vi "PPG_ABC.calc temp pattern.vi"(0 "i ref in":refnum<vi>, 2 "PGData":T3, 4 "clockRate [ticks/us]":dbl, 5 "error in (no error)":errorcluster) -> (14 "i ref out":refnum<vi>, 16 "patternDefs":T2(array[cluster]), 19 "error out":errorcluster)   [LabVIEW 2014, in "PPG_ABC.lvlib"]
doc: "Calculates the pattern definition array. This method starts from a public pattern format defined by this class and converts it into an intermediate pattern definition array."
uses:
  PPG_ABC.lvlib
  PPG_ABC.PG_dataType.ctl
  CS_Core/CSSystem/CoreDefs/CoreDefs.error_type.ctl
  CS_Core/CSSystem/CoreDefs/CoreDefs.error_severity.ctl
  CS_Core/CSSystem/CoreLib/CoreLib.lvlib
panel:
  in  "patternDef":T1
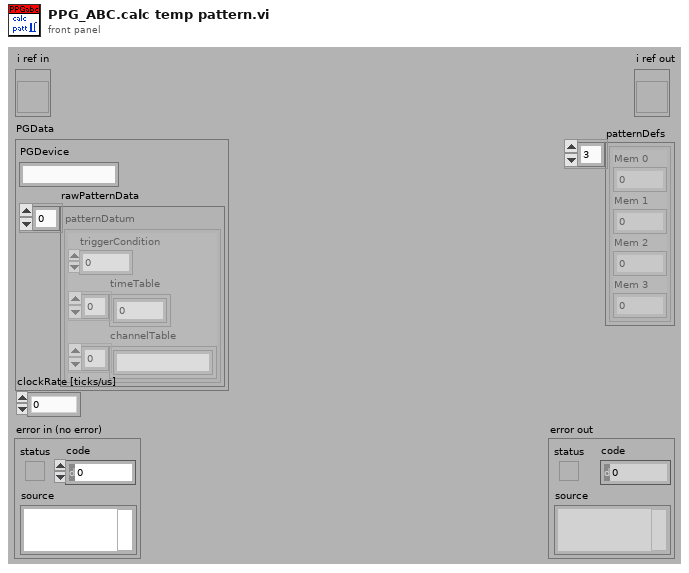
[diagram p1: front panel]
types:
  T1 = cluster{"Mem 0":u8, "Mem 1":u32, "Mem 2":u32, "Mem 3":u32}
  T2 = cluster{"Mem 0":u8, "Mem 1":u32, "Mem 2":u32, "Mem 3":u32}[]
  T3 = typedef "PPG_ABC.lvlib/PPG_ABC.PG_dataType.ctl" = cluster{"PGDevice":string, "rawPatternData":cluster{"triggerCondition":i32, "timeTable":dbl[], "channelTable":string[]}[]}
  T4 = typedef "CoreDefs.error_severity.ctl" = enum16{"undefined", "information", "warning", "error", "fatal"}
  T5 = typedef "CoreDefs.error_type.ctl" = enum16{"no error", "can't load process", "can't unload process", "process does not exist", "can't install process", "can't remove process", "unknown function", "time out", "can't execute function", "duplicate queue name", "super not found", "caller queue invalid", "can't ping process", "unknown error", "VISA Error", "VISA timeout", "GPIB timeout", "GPIB error", "communication error", "data type mismatch", "can't read data from OPC server", "can't write data to OPC server", "OET error", "function not implemented", "process already exists", "invalid Shared Variable name", "error writing Shared Variable", "error reading Shared Variable", "invalid client name", "corrupt database", "unknown class", "call not authorized", "parameter out of range", "OET timeout: can't get data to modify", "invalid queue name", "requested operation incompatible with current state", "event undefined", "event disabled", "state undefined", "caller is not a friend", "EventBuilder: bad eventID", "EventBuilder: no DAQ devices", "a thread must not stop itself", "UNUSED ELEMENT4", "DiscArchiver: eventData incomplete", "DiscArchiver: eventData does not belong to run", "DiscArchiver: can't open file", "DiscArchiver: can't write to file", "DiscArchiver: available disc space low", "can't acquire semaphore", "error reading data from database", "notifier object is not existing", "can't register process", "can't unregister process", "illegal event type", "object disabled", "object already exists", "can't change state", "Instrument not found", "no connection to remote node", "invalid reference", "N/A", "UNUSED ELEMENT 1", "element not found", "illegal TCP/IP connection detected", "object does not exist", "invalid access ID", "unknown CS system", "invalid privilige", "unsupported data type", "unsupported server type", "IO server already exists", "Shared Variable already exists"}
  T6 = cluster{"triggerCondition":i32, "timeTable":dbl[], "channelTable":string[]}[]
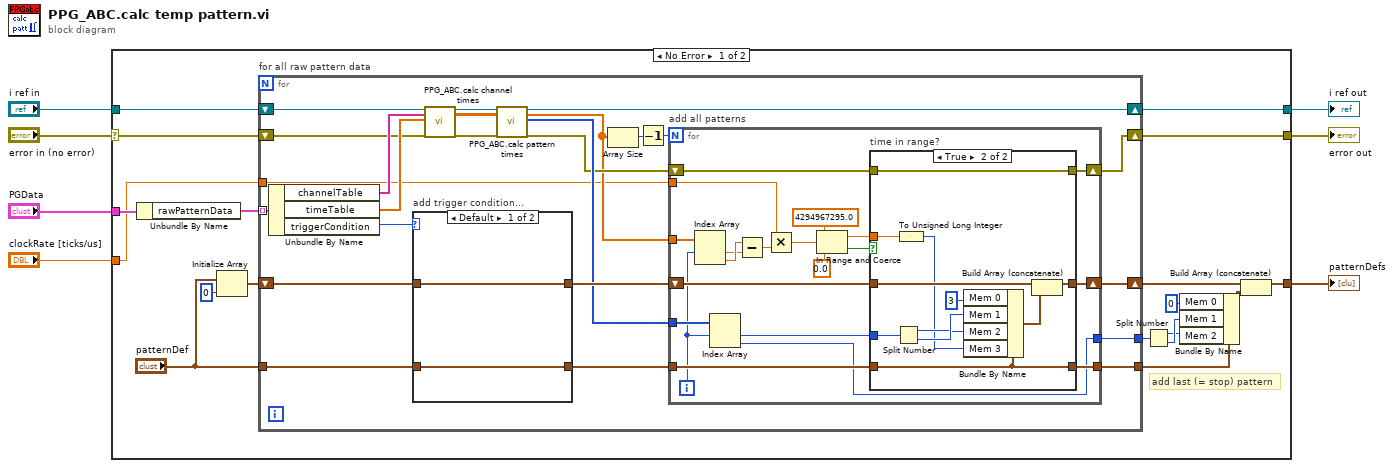
[diagram p0: block diagram]
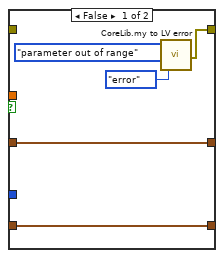
[diagram p2: hidden frame]
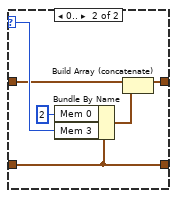
[diagram p3: hidden frame]
diagram:
  n1 = case shown="No Error" "error in (no error)" {
    selector: "error in (no error)" -> [w8 w94]
    tunnel: "i ref in" -> [w9 w95]
    tunnel: [w15 w95] -> w6
    tunnel: [w14 w94] -> w5
    tunnel: "PGData" -> [w25 _]
    tunnel: [w16 _] -> w2
    tunnel: "clockRate [ticks/us]" -> [w10 _]
    frame No Error {
      # "add last (= stop) pattern"
      n2 = Unbundle By Name(w25) -> ("rawPatternData"=w24:T6)
      n3 = Initialize Array("patternDef", 0 ("dimension size")) -> (w21:T2)
      n4 = for "for all raw pattern data" {
        tunnel: w24 -> [w49] mode=indexing
        shift-right: [w34] -> w17
        shift-left: w21 -> [w46]
        tunnel: "patternDef" -> [w47]
        shift-right: [w36] -> w15
        shift-left: w9 -> [w27]
        shift-right: [w35] -> w14
        shift-left: w8 -> [w28]
        tunnel: [w33] -> w20
        tunnel: [w29] -> w11
        tunnel: w10 -> [w26]
        n5 = Unbundle By Name(w49) -> ("channelTable"=w45:string[], "timeTable"=w44:dbl[], "triggerCondition"=w48:i32)
        n6 = case "add trigger condition..." shown="Default" w48 {
          selector: w48 -> [_ w93]
          tunnel: w47 -> [w86 w88]
          tunnel: w46 -> [w87 w91]
          tunnel: [w87 w89] -> w40
          tunnel: [w86 w88] -> w38
          frame Default {
          }
          frame 0.. {
            n7 = Bundle By Name(cluster=w88, "Mem 0"=u8 2, "Mem 3"=w93) -> (w90:T1)
            n8 = Build Array (concatenate)(w91, w90) -> (w89:T2)
          }
        }
        n9 = call "PPG_ABC.calc channel times.vi"("i ref in"=w27, "channelTable"=w45, "timeTable"=w44, "error in (no error)"=w28) -> ("i ref out"=w42:refnum<vi>, "channelTimes"=w41:dbl[][], "error out"=w43:errorcluster)  [unwired: 13 in]
        n10 = call "PPG_ABC.calc pattern times.vi"("i ref in"=w42, "channelTimes"=w41, "error in (no error)"=w43) -> ("i ref out"=w36:refnum<vi>, "patternTimes"=w31:dbl[], "patterns"=w39:u64[], "error out"=w37:errorcluster)  [unwired: 13 in]
        n11 = Array Size(array=w31) -> (size(s)=w32:i32)
        n12 = Decrement(x=w32) -> (x-1=w30:i32)
        n13 = for "add all patterns" {
          N: w30 -> [_]
          shift-right: [w68] -> w34
          shift-left: w40 -> [w69]
          tunnel: w31 -> [w65]
          tunnel: w38 -> [w67]
          tunnel: w39 -> [w66]
          shift-right: [w55] -> w35
          shift-left: w37 -> [w56]
          tunnel: [w54] -> w33
          tunnel: [w51] -> w29
          tunnel: w26 -> [w50]
          i -> [w52]
          n14 = Index Array(array=w65, index #1=w52) -> (element #1=w63:dbl, element #2=w64:dbl)  [unwired: 1 in]
          n15 = Index Array(array=w66, index #1=w52) -> (element #1=w53:u64, element #2=w51:u64)  [unwired: 1 in]
          n16 = Subtract(x=w64, y=w63) -> (x-y=w62:dbl)
          n17 = Multiply(x=w50, y=w62) -> (x*y=w61:dbl)
          n18 = In Range and Coerce(upper limit=4294967295.0, x=w61, lower limit=0.0) -> (coerced(x)=w58:dbl, In Range?=w57:bool)
          n19 = case "time in range?" shown="True" w57 {
            tunnel: w69 -> [w74 w83]
            tunnel: [w74 w82] -> w68
            tunnel: w67 -> [w70 w75]
            tunnel: w53 -> [_ w81]
            tunnel: w58 -> [_ w77]
            tunnel: w56 -> [_ w76]
            tunnel: [w73 w76] -> w55
            tunnel: [w70 w75] -> w54
            frame False {
              n20 = call "CoreLib.my to LV error.vi"("ErrorTypes"=CoreDefs.error_type."parameter out of range", "severityLevel"=CoreDefs.error_severity."error") -> ("myErrorCluster"=w73:errorcluster)  [unwired: 16 in, 1 out]
            }
            frame True {
              n21 = Split Number(x=w81) -> (hi(x)=w79:u32, lo(x)=w80:u32)
              n22 = To Unsigned Long Integer(number=w77) -> (unsigned 32bit integer=w78:u32)
              n23 = Bundle By Name(cluster=w75, "Mem 0"=u8 3, "Mem 1"=w80, "Mem 2"=w79, "Mem 3"=w78) -> (w85:T1)
              n24 = Build Array (concatenate)(w83, w85) -> (w82:T2)
            }
          }
        }
      }
      n25 = Split Number(x=w11) -> (hi(x)=w12:u32, lo(x)=w13:u32)
      n26 = Bundle By Name(cluster=w20, "Mem 0"=u8 0, "Mem 1"=w13, "Mem 2"=w12) -> (w18:T1)
      n27 = Build Array (concatenate)(w17, w18) -> (w16:T2)
    }
    frame Error {
    }
  }
  "error out" <- w5
  "i ref out" <- w6
  "patternDefs" <- w2
